vi "SetSplittersWidths.vi"(8 "error in (no error)":errorcluster, 11 "Splitters":T2) -> (0 "error out":errorcluster, 3 "Splitters Widths":T1)   [LabVIEW 2022 SP3, in "PentaPanesLibrary.lvlib" / "PentaPanes.lvclass"]
uses:
  PentaPanes.lvclass
  SplittersWidthCluster.ctl
  SplittersCluster.ctl
panel:
  in  "Splitters Widths 2":T1={"Top Splitter"=2, "Left Splitter"=2, "Right Splitter"=2, "Bottom Splitter"=2}
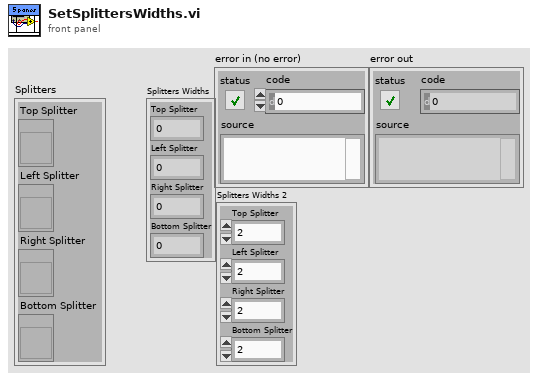
[diagram p1: front panel]
types:
  T1 = typedef "PentaPanesLibrary.lvlib/PentaPanes.lvclass/SplittersWidthCluster.ctl" = cluster{"Top Splitter":i32, "Left Splitter":i32, "Right Splitter":i32, "Bottom Splitter":i32}
  T2 = typedef "PentaPanesLibrary.lvlib/PentaPanes.lvclass/SplittersCluster.ctl" = cluster{"Top Splitter":refnum<vi>, "Left Splitter":refnum<vi>, "Right Splitter":refnum<vi>, "Bottom Splitter":refnum<vi>}
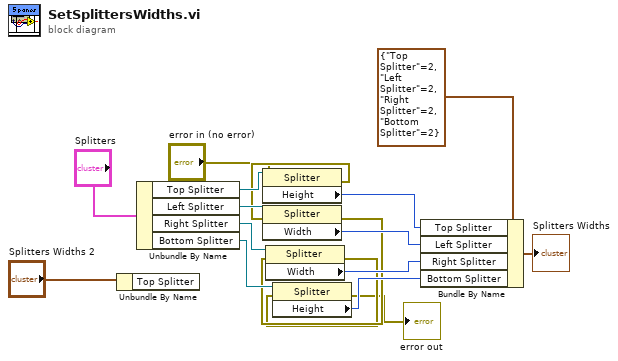
[diagram p0: block diagram]
diagram:
  n1 = Unbundle By Name("Splitters Widths 2") -> ()  [unwired: 1 out]
  n2 = Unbundle By Name("Splitters") -> ("Top Splitter"=w9:refnum<vi>, "Left Splitter"=w11:refnum<vi>, "Right Splitter"=w12:refnum<vi>, "Bottom Splitter"=w10:refnum<vi>)
  n3 = property class="Splitter"(reference=w9, error in="error in (no error)") -> (error out=w7:errorcluster, "Height"=w1:u32)  [unwired: 1 out]
  n4 = property class="Splitter"(reference=w11, error in=w7) -> (error out=w6:errorcluster, "Width"=w13:u32)  [unwired: 1 out]
  n5 = property class="Splitter"(reference=w12, error in=w6) -> (error out=w5:errorcluster, "Width"=w14:u32)  [unwired: 1 out]
  n6 = property class="Splitter"(reference=w10, error in=w5) -> (error out=→"error out":errorcluster, "Height"=w15:u32)  [unwired: 1 out]
  n7 = Bundle By Name(cluster=T1 {"Top Splitter"=2, "Left Splitter"=2, "Right Splitter"=2, "Bottom Splitter"=2} ("Splitters Widths"), "Top Splitter"=w1, "Left Splitter"=w13, "Right Splitter"=w14, "Bottom Splitter"=w15) -> (→"Splitters Widths":T1)
